vi "BenchmarkLocalize.vi"() -> ()   [LabVIEW 2011]
uses:
  TrackerVIs/TrackerDLL.vi
panel:
  in  "Show traces?":bool
  out "FPS":dbl
  out "Loop count":i32
  out "appended path":path
  in  "Show graphs":bool
  in  "Use debug library":bool
  in  "xcor_iterations":i32=2
  out "X profile":sgl[](graph)
  out "Y profile":sgl[](graph)
  out "Y result":sgl[](graph)
  out "True Y":dbl
  out "True X":dbl
  out "COM results":cluster{dbl, dbl}(graph)
  out "XCor results":cluster{dbl, dbl}(graph)
  in  "y center":dbl=75.0
  in  "x center":dbl=75.0 min=40.0 max=200.0
  out "X result":sgl[](graph)
  in  "spotsize":sgl=2.0 min=1 max=20
  in  "Stop loop":bool
  out "median":sgl
  out "xcorpos":cluster{"XCor X":sgl, "XCor Y":sgl}
  out "COM":cluster{"comX":sgl, "comY":sgl}
  out "Image":T1(plugin-control)
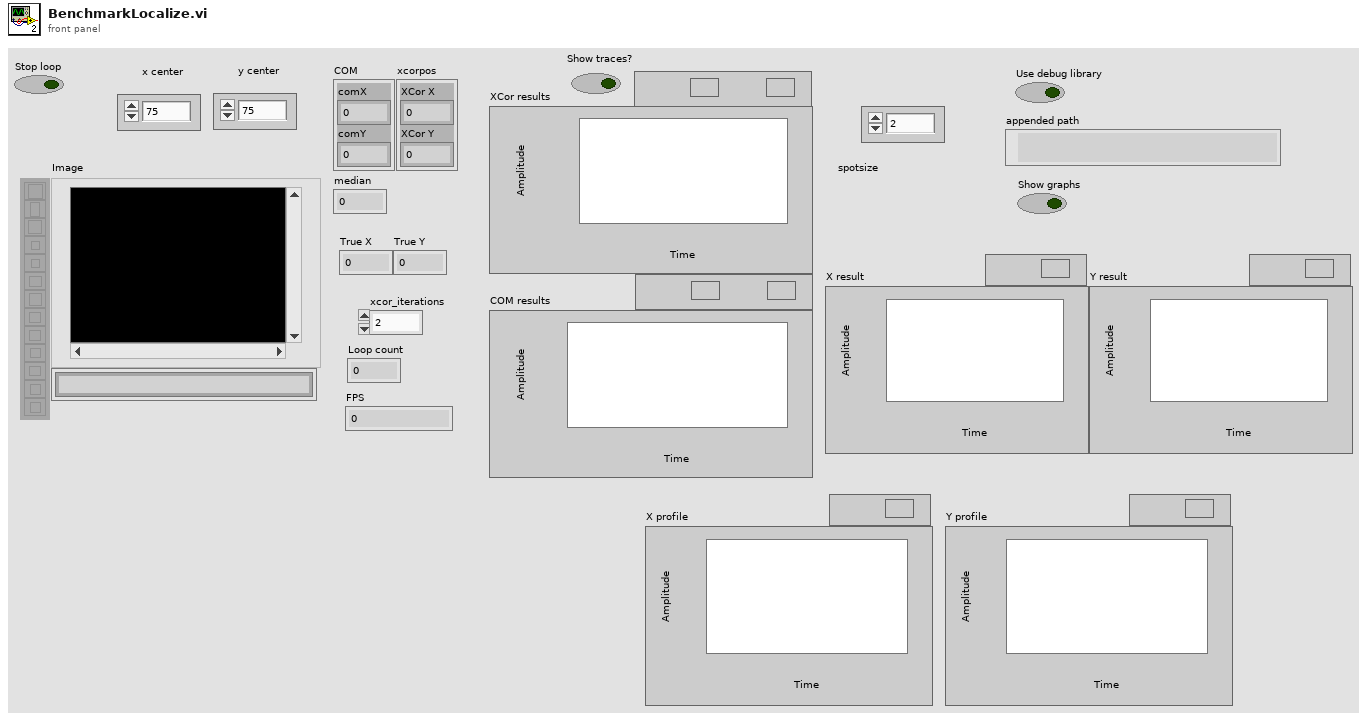
[diagram p1: front panel]
types:
  T1 = typedef "IMAQ Image.ctl" = refnum<image>
  T2 = typedef "Image Type" = u32
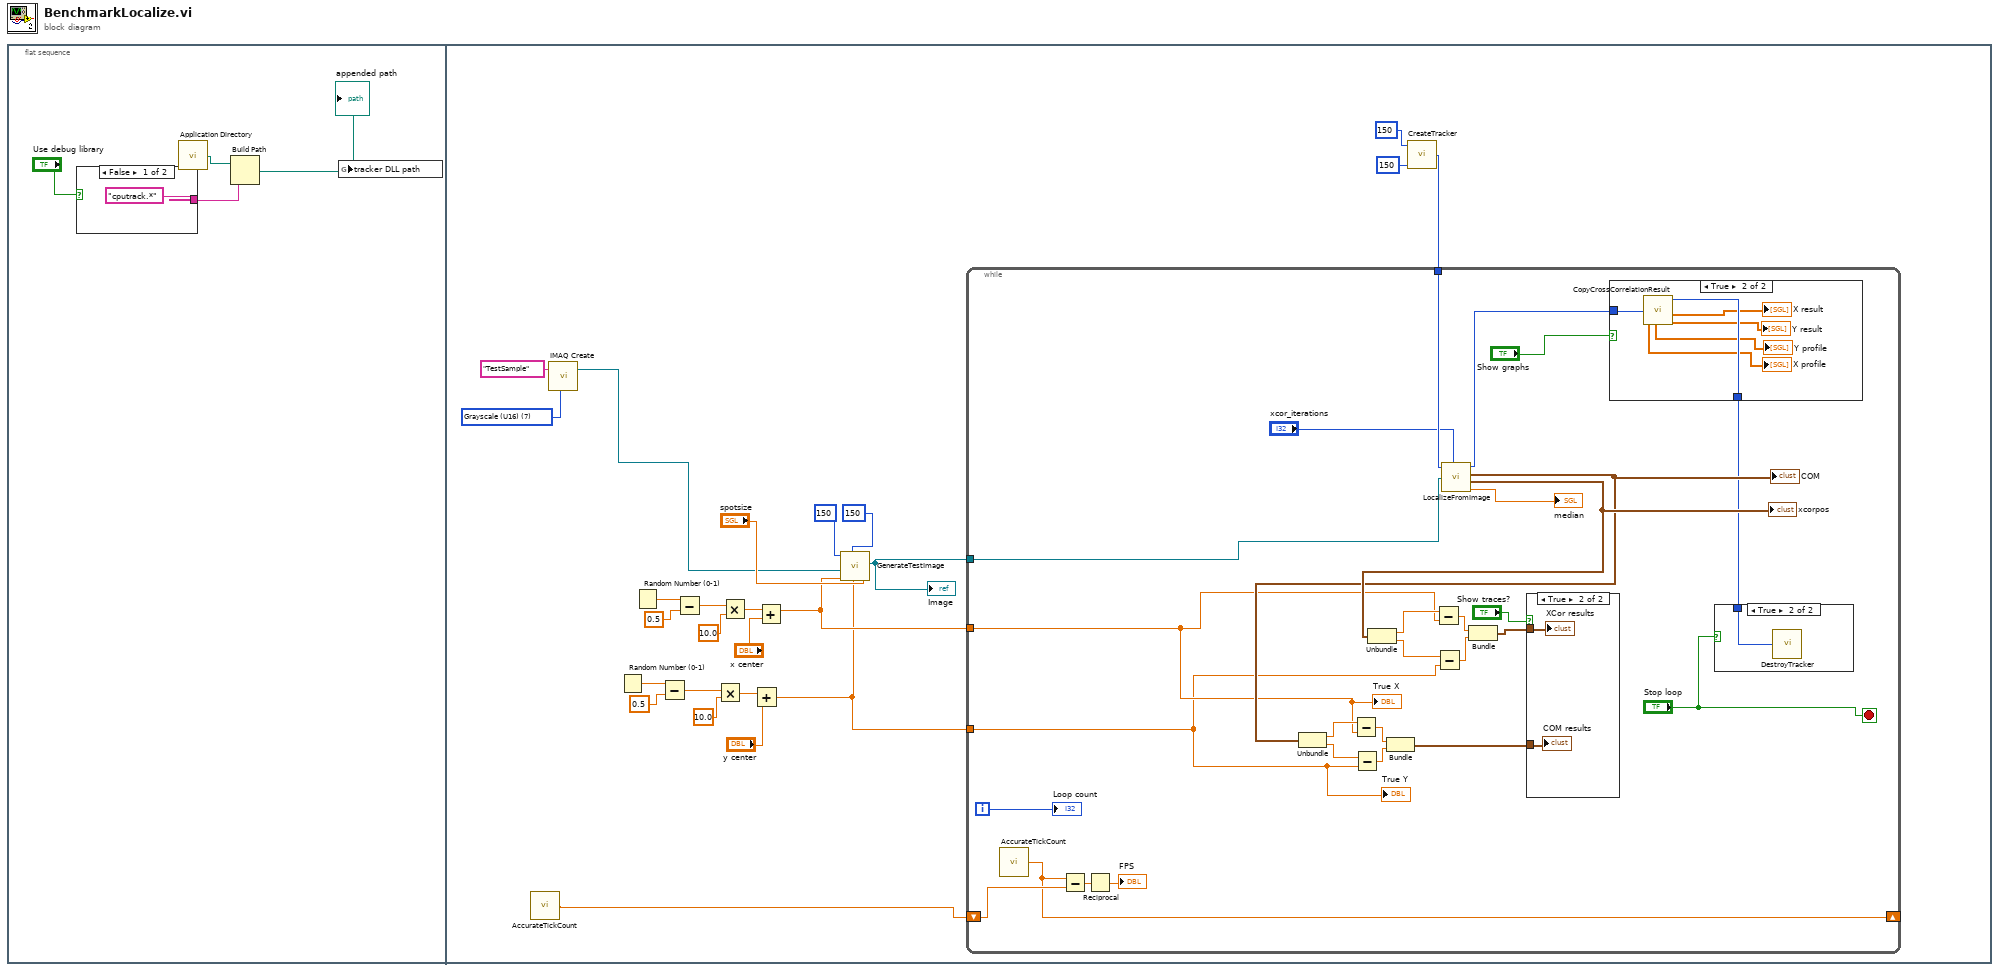
[diagram p0: block diagram]
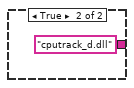
[diagram p2: hidden frame]
diagram:
  n1 = flat-sequence {
    frame #0 {
      n2 = case shown="False" "Use debug library" {
        tunnel: ["cputrack.*" "cputrack_d.dll"] -> w2
        frame False {
        }
        frame True {
        }
      }
      n3 = call <vilib>:"Application Directory.vi"() -> ("Application Directory"=w1:path)
      n4 = Build Path(base path=w1, name or relative path=w2) -> (appended path=w3:path)
      "appended path" <- w3
      n5 = global write "TrackerDLL.vi" "tracker DLL path"(w3) -> ()
    }
    frame #1 {
      w31 = T2 7 items=["Grayscale (U8)", "Grayscale (I16)", "Grayscale (SGL)", "Complex (CSG)", "RGB (U32)", "HSL (U32)", "RGB (U64)", "Grayscale (U16)"] ("Image Type")
      n6 = call "AccurateTickCount.vi"() -> ("seconds"=w26:dbl)
      n7 = call "IMAQ Create"("Image Name"="TestSample" ("String"), "Image Type"=w31) -> ("New Image"=w8:T1)  [unwired: 3 in, 1 out]
      n8 = Random Number (0-1)() -> (number: 0 to 1=w23:dbl)
      n9 = Random Number (0-1)() -> (number: 0 to 1=w19:dbl)
      n10 = Subtract(x=w23, y=0.5) -> (x-y=w25:dbl)
      n11 = Subtract(x=w19, y=0.5) -> (x-y=w22:dbl)
      n12 = Multiply(x=w25, y=sgl 10.0) -> (x*y=w16:dbl)
      n13 = Multiply(x=w22, y=sgl 10.0) -> (x*y=w14:dbl)
      n14 = Add(x=w16, y="y center") -> (x+y=w9:dbl)
      n15 = Add(x=w14, y="x center") -> (x+y=w10:dbl)
      n16 = call "GenerateTestImage.vi"("spotsize"="spotsize", "ypos"=w9, "height"=u32 150, "xpos"=w10, "image"=w8, "width"=u32 150) -> ("Image"=w7:T1)  [unwired: 3 in]
      "Image" <- w7
      n17 = call "CreateTracker.vi"("height"=u32 150, "width"=u32 150) -> ("return type"=w29:u64)  [unwired: 1 in]
      n18 = while {
        tunnel: w29 -> [w59]
        shift-right: [w39] -> _
        shift-left: w26 -> [w40]
        tunnel: w10 -> [w36]
        tunnel: w9 -> [w35]
        tunnel: w7 -> [w34]
        i -> [w41]
        stop <- "Stop loop" stop-if-true
        n19 = call "AccurateTickCount.vi"() -> ("seconds"=w39:dbl)
        n20 = Subtract(x=w39, y=w40) -> (x-y=w38:dbl)
        n21 = Reciprocal(x=w38) -> (1/x=→"FPS":dbl)
        n22 = call "LocalizeFromImage.vi"("tracker"=w59, "xcor_iterations"="xcor_iterations", "input image"=w34) -> ("tracker"=w45:u64, "COM"=w48:cluster{"comX":sgl, "comY":sgl}, "xcorpos"=w56:cluster{"XCor X":sgl, "XCor Y":sgl}, "median"=→"median":sgl)  [unwired: 4 in]
        "COM" <- w48
        "xcorpos" <- w56
        n23 = Unbundle(w48) -> ("comX"=w47:sgl, "comY"=w46:sgl)
        n24 = Subtract(x=w47, y=w36) -> (x-y=w50:dbl)
        n25 = Subtract(x=w46, y=w35) -> (x-y=w49:dbl)
        n26 = Unbundle(w56) -> ("XCor X"=w55:sgl, "XCor Y"=w54:sgl)
        n27 = Bundle(w50, w49) -> (w33:cluster{dbl, dbl})  [unwired: 1 in]
        n28 = Subtract(x=w55, y=w36) -> (x-y=w53:dbl)
        n29 = Subtract(x=w54, y=w35) -> (x-y=w52:dbl)
        n30 = Bundle(w53, w52) -> (w51:cluster{dbl, dbl})  [unwired: 1 in]
        n31 = case shown="True" "Show traces?" {
          tunnel: w51 -> [_ w61]
          tunnel: w33 -> [_ w60]
          frame False {
          }
          frame True {
            "XCor results" <- w61
            "COM results" <- w60
          }
        }
        n32 = case shown="True" "Show graphs" {
          tunnel: w45 -> [w62 w68]
          tunnel: [w62 w67] -> w44
          frame False {
          }
          frame True {
            n33 = call "CopyCrossCorrelationResult.vi"("tracker"=w68) -> ("x prof"=→"X profile":sgl[], "y prof"=→"Y profile":sgl[], "tracker"=w67:u64, "x result"=→"X result":sgl[], "y_result"=→"Y result":sgl[])  [unwired: 3 in]
          }
        }
        n34 = case shown="True" "Stop loop" {
          tunnel: w44 -> [_ w69]
          frame False {
          }
          frame True {
            n35 = call "DestroyTracker.vi"("tracker"=w69) -> ()
          }
        }
        "True X" <- w36
        "True Y" <- w35
        "Loop count" <- w41
      }
    }
  }
